vi "command identifier.vi"(11 "Input command":string="Write to VISA, \u0000\u0000\u0000\u000eGPIB::12::inst, , offoff") -> (3 "Identifield command":string="Write to VISA")   [LabVIEW 2019]
panel:
  out "param dep.":i32[](array[numeric])=[-1, -1, -1]
  out "stand alone":i32[](array[numeric])=[-1, -1, -1, -1, -1, -1, -1, -1, -1, -1, -1, -1, -1, -1, -1, -1, -1, 2017, -1]
  in  "param dependent command":string[](array[string])=["dummy", "Set", "Wait for"]
  in  "stand alone commands":string[](array[string])=["Set Field", "Set Temperature", "Sweep", "Start", "Stop", "Wait for Temperature", "Wait for Field Stable", "Wait for VI value", "Remarks", "----------", "Run VI", "Abort VI", "Set Parameter", "Wait for MPMS trigger", "Run Macro", "END SUBsequence", "SubMacro", "Write to VISA", "END SEQUENCE"]
  in  "command list-all":string[](array[string])=["Set Field", "Set Temperature", "Set", "Sweep", "Start", "Stop", "Wait for", "Wait for Temperature", "Wait for Field Stable", "Wait for VI value", "Set Parameter", "Remarks", "----------", "Run VI", "Abort VI", "Wait for MPMS trigger", "Run Macro", "END SUBsequence", "SubMacro", "Write to VISA", "END SEQUENCE"]
  # "Identifies the command in the sequence and assign a command identifier in the que.\nEach identifier will determine the next action.\nNote there are two types of command (stand-alone and parameter-dependent). \nA third type command (skip, remark) also exist, which are dealt with separately inside the code."
  # "Commands that requires parameters."
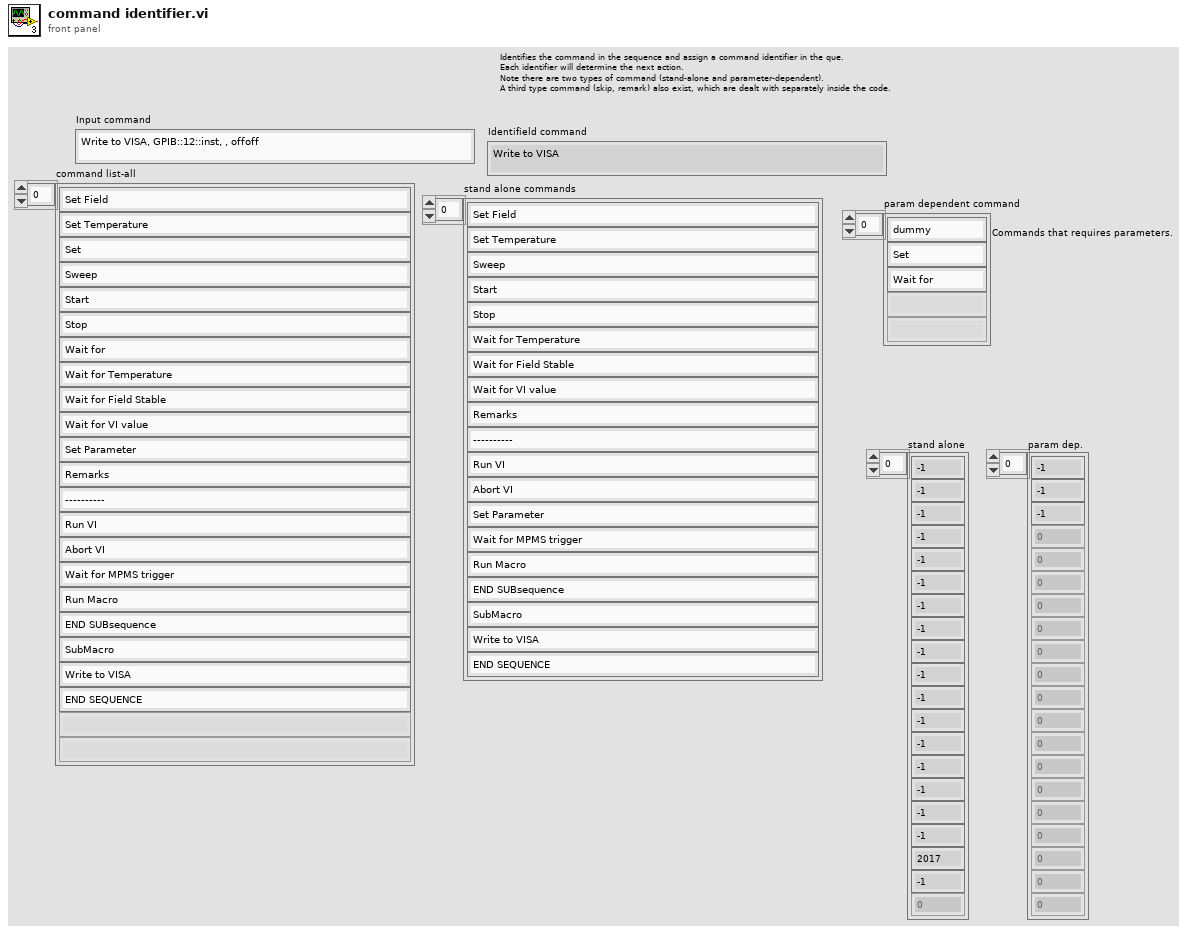
[diagram p1: front panel]
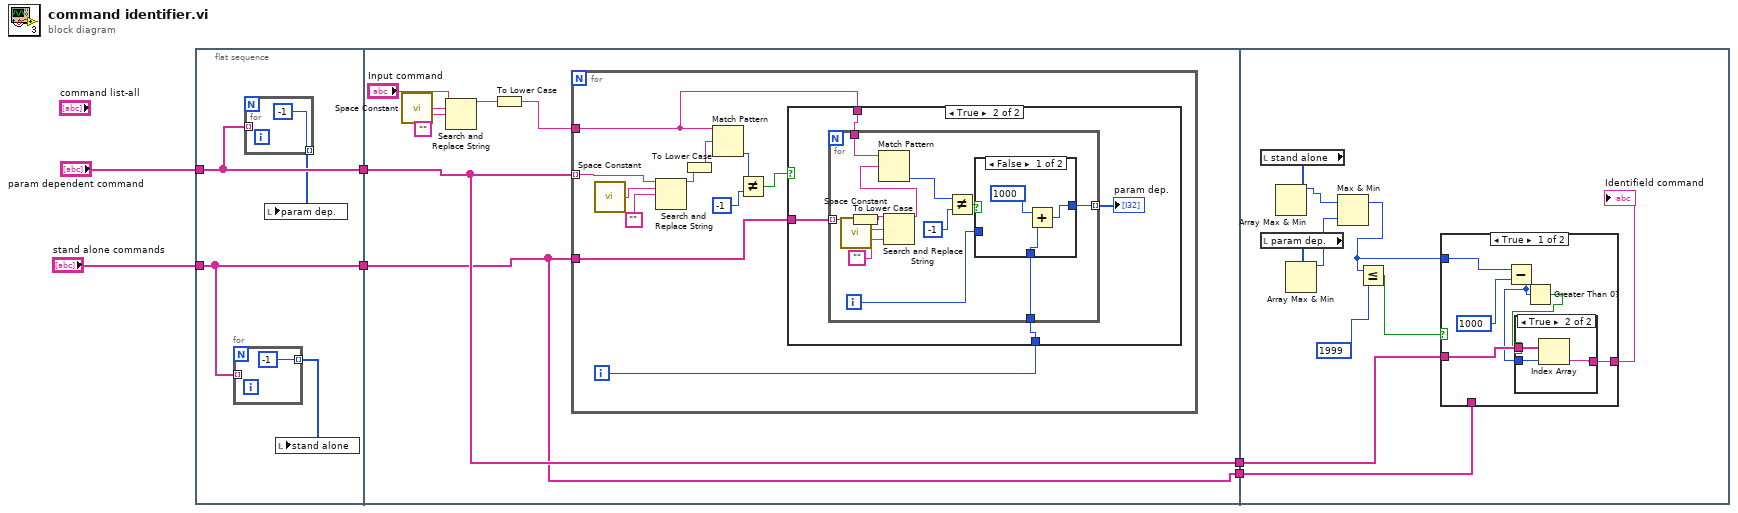
[diagram p0: block diagram]
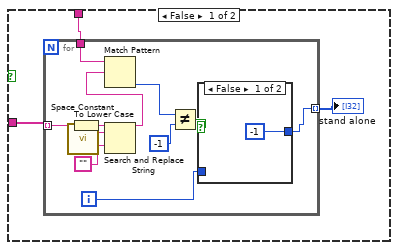
[diagram p2: hidden frame]
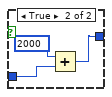
[diagram p3: hidden frame]
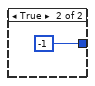
[diagram p4: hidden frame]
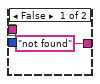
[diagram p5: hidden frame]
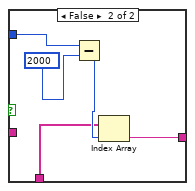
[diagram p6: hidden frame]
diagram:
  n1 = flat-sequence {
    tunnel: [w10] -> w4
    tunnel: "param dependent command" -> [w10]
    tunnel: [w9] -> w2
    tunnel: "stand alone commands" -> [w9]
    tunnel: [w14] -> w6
    tunnel: [w13] -> w5
    tunnel: w4 -> [w14]
    tunnel: w2 -> [w13]
    tunnel: w6 -> [w72]
    tunnel: w5 -> [w69]
    frame #0 {
      n2 = for {
        tunnel: w9 -> [_] mode=indexing
        tunnel: [-1] -> w8 mode=indexing
      }
      n3 = for {
        tunnel: w10 -> [_] mode=indexing
        tunnel: [-1] -> w7 mode=indexing
      }
      n4 = local write "param dep."(w7) -> ()
      n5 = local write "stand alone"(w8) -> ()
    }
    frame #1 {
      n6 = call <vilib>:"Space Constant.vi"() -> ("String"=w19:string)
      n7 = Search and Replace String(input string="Input command", search string=w19, replace string="") -> (result string=w17:string)  [unwired: 5 in, 3 out]
      n8 = To Lower Case(string=w17) -> (all lower case string=w16:string)
      n9 = for {
        tunnel: w16 -> [w24]
        tunnel: w14 -> [w22] mode=indexing
        tunnel: w13 -> [w20]
        i -> [w21]
        n10 = call <vilib>:"Space Constant.vi"() -> ("String"=w30:string)
        n11 = Search and Replace String(input string=w22, search string=w30, replace string="") -> (result string=w28:string)  [unwired: 5 in, 3 out]
        n12 = To Lower Case(string=w28) -> (all lower case string=w23:string)
        n13 = Match Pattern(string=w24, regular expression=w23) -> (offset past match=w27:i32)  [unwired: 1 in, 3 out]
        n14 = Not Equal?(x=w27, y=-1) -> (x != y?=w25:bool)
        n15 = case shown="True" w25 {
          tunnel: w24 -> [w33 w52]
          tunnel: w20 -> [w32 w51]
          tunnel: w21 -> [_ w50]
          frame False {
            n16 = for {
              tunnel: w32 -> [w36] mode=indexing
              tunnel: w33 -> [w41]
              tunnel: [w34] -> w31 mode=indexing
              i -> [w35]
              n17 = call <vilib>:"Space Constant.vi"() -> ("String"=w43:string)
              n18 = To Lower Case(string=w36) -> (all lower case string=w37:string)
              n19 = Search and Replace String(input string=w37, search string=w43, replace string="") -> (result string=w42:string)  [unwired: 5 in, 3 out]
              n20 = Match Pattern(string=w41, regular expression=w42) -> (offset past match=w38:i32)  [unwired: 1 in, 3 out]
              n21 = Not Equal?(x=w38, y=-1) -> (x != y?=w39:bool)
              n22 = case shown="False" w39 {
                tunnel: [-1 ("y") w47] -> w34
                tunnel: w35 -> [_ w48]
                frame False {
                }
                frame True {
                  n23 = Add(x=2000, y=w48) -> (x+y=w47:i32)
                }
              }
            }
            "stand alone" <- w31
          }
          frame True {
            n24 = for {
              tunnel: w51 -> [w55] mode=indexing
              tunnel: w52 -> [w61]
              tunnel: w50 -> [w54]
              tunnel: [w53] -> w49 mode=indexing
              i -> [w56]
              n25 = call <vilib>:"Space Constant.vi"() -> ("String"=w63:string)
              n26 = To Lower Case(string=w55) -> (all lower case string=w57:string)
              n27 = Search and Replace String(input string=w57, search string=w63, replace string="") -> (result string=w62:string)  [unwired: 5 in, 3 out]
              n28 = Match Pattern(string=w61, regular expression=w62) -> (offset past match=w59:i32)  [unwired: 1 in, 3 out]
              n29 = Not Equal?(x=w59, y=-1) -> (x != y?=w58:bool)
              n30 = case shown="False" w58 {
                tunnel: w56 -> [_ _]
                tunnel: [w67 -1 ("y")] -> w53
                tunnel: w54 -> [w66 _]
                frame False {
                  n31 = Add(x=1000, y=w66) -> (x+y=w67:i32)
                }
                frame True {
                }
              }
            }
            "param dep." <- w49
          }
        }
      }
    }
    frame #2 {
      n32 = local read "stand alone"() -> (w78:i32[])
      n33 = local read "param dep."() -> (w77:i32[])
      n34 = Array Max & Min(array=w78) -> (max value=w76:i32)  [unwired: 3 out]
      n35 = Array Max & Min(array=w77) -> (max value=w75:i32)  [unwired: 3 out]
      n36 = Max & Min(x=w76, y=w75) -> (max(x,y)=w71:i32)  [unwired: 1 out]
      n37 = Less Or Equal?(x=w71, y=1999) -> (x <= y?=w73:bool)
      n38 = case shown="True" w73 {
        tunnel: w72 -> [w84 _]
        tunnel: w71 -> [w83 w93]
        tunnel: [w81 w90] -> w70
        tunnel: w69 -> [_ w89]
        frame True {
          n39 = Subtract(x=w83, y=1000) -> (x-y=w79:i32)
          n40 = Greater Than 0?(x=w79) -> (x > 0?=w80:bool)
          n41 = case shown="True" w80 {
            tunnel: w84 -> [_ w88]
            tunnel: ["not found" ("String") w87] -> w81
            tunnel: w79 -> [_ w86]
            frame False {
            }
            frame True {
              n42 = Index Array(array=w88, index=w86) -> (element=w87:string)
            }
          }
        }
        frame False {
          n43 = Subtract(x=w93, y=2000) -> (x-y=w91:i32)
          n44 = Index Array(array=w89, index=w91) -> (element=w90:string)
        }
      }
      "Identifield command" <- w70
    }
  }
